vi "Do.vi"(8 "error in (no error)":errorcluster, 10 "Actor in":refnum<class "Actor.lvclass">, 11 "Enqueue Logs Element Msg":refnum<class "Enqueue Logs Element Msg.lvclass">) -> (0 "error out":errorcluster, 2 "Actor out":refnum<class "Actor.lvclass">)   [LabVIEW 2019, in "EventLog.lvlib" / "Enqueue Logs Element Msg.lvclass"]
doc: "This VI delivers the message to the actor by calling the appropriate method(s) on the actor."
uses:
  Enqueue Logs Element Msg.lvclass
  EventLog/EventLog.lvclass
  Classes/Event/Event.lvclass
  Obtain and Save Msg/Obtain and Save Msg.lvclass
  <vilib>/ActorFramework/Actor/Actor.lvclass
  C:/Projekty/_Wewnetrzne/PC_ActorFramework/07_Program/LABVIEW/02_Source/Classes/EventsAbstract/EventsAbstract.lvclass
  C:/Projekty/_Wewnetrzne/PC_ActorFramework/07_Program/LABVIEW/02_Source/SubModules/LogsAbstract/LogsAbstract.lvclass
  C:/Projekty/_Wewnetrzne/PC_ActorFramework/07_Program/LABVIEW/02_Source/Modules/ModuleAbstract/ModuleAbstract.lvclass
  C:/Program Files (x86)/National Instruments/LabVIEW 2019/vi.lib/MGI/Monitored Actor/Monitored Actor/Monitored Actor/Monitored Actor.lvclass
  C:/Program Files (x86)/National Instruments/LabVIEW 2019/vi.lib/ActorFramework/Actor/Actor.lvclass
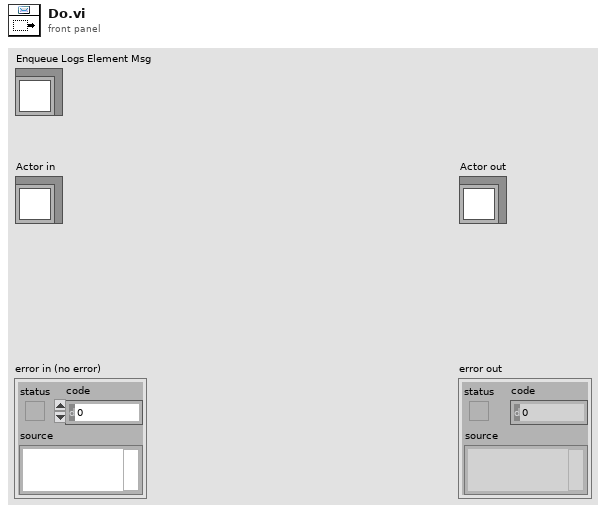
[diagram p1: front panel]
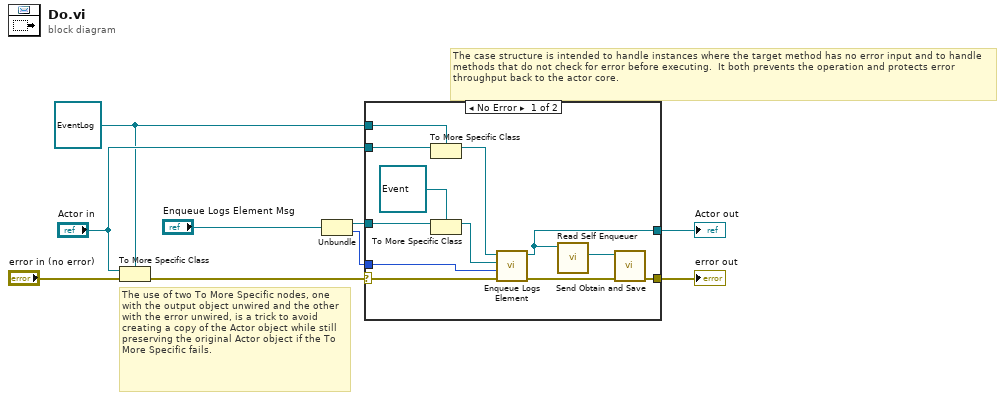
[diagram p0: block diagram]
diagram:
  w3 = refnum<class "EventLog.lvclass"> refnum ("Actor in")
  # "The use of two To More Specific nodes, one with the output object unwired and the other with the error unwired, is a trick to avoid creating a copy of the Actor object while still preserving the original Actor object if the To More Specific fails."
  # "The case structure is intended to handle instances where the target method has no error input and to handle methods that do not check for error before executing.  It both prevents the operation and protects error throughput back to the actor core."
  n1 = To More Specific Class(target class=w3, reference="Actor in", error in="error in (no error)") -> (error out=w7:errorcluster)  [unwired: 1 out]
  n2 = Unbundle("Enqueue Logs Element Msg") -> (w2:refnum<class "EventsAbstract.lvclass">, w1:i32)
  n3 = case shown="No Error" w7 {
    selector: w7 -> [w21 w23]
    tunnel: [w12 w23] -> w6
    tunnel: [w11 w22] -> w5
    tunnel: "Actor in" -> [w20 w22]
    tunnel: w3 -> [w19 _]
    tunnel: w2 -> [w15 _]
    tunnel: w1 -> [w17 _]
    frame No Error {
      n4 = To More Specific Class(target class=w19, reference=w20) -> (specific class reference=w18:refnum<class "EventLog.lvclass">)  [unwired: 1 in, 1 out]
      n5 = To More Specific Class(target class=refnum<class "Event.lvclass"> refnum ("Event.lvclass"), reference=w15) -> (specific class reference=w16:refnum<class "Event.lvclass">)  [unwired: 1 in, 1 out]
      n6 = call-dynamic "Enqueue Logs Element.vi"("Error In"=w21, "Timeout"=w17, "Event Occured"=w16, "EventLog in"=w18) -> ("Error Out"=w13:errorcluster, "EventLog out"=w11:refnum<class "EventLog.lvclass">)  [unwired: 5 in, 1 out]
      n7 = call <vilib>:"Read Self Enqueuer.vi"("Actor"=w11) -> ("Self Enqueuer"=w10:refnum<class "Message Enqueuer.lvclass">)  [unwired: 10 in]
      n8 = call "Send Obtain and Save.vi"("error in (no error)"=w13, "Message Enqueuer"=w10) -> ("error out"=w12:errorcluster)  [unwired: 8 in, 1 out]
    }
    frame Error {
      # "If type check fails, pass the original object out again."
    }
  }
  "error out" <- w6
  "Actor out" <- w5
